vi "data2string.vi"(1 "Units":string="A", 2 "Numeric":dbl=0.0999646 format="%#_6p") -> (0 "resulting string":string="  99.964600   mA")   [LabVIEW 2013]
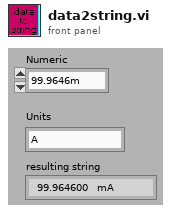
[diagram p1: front panel]
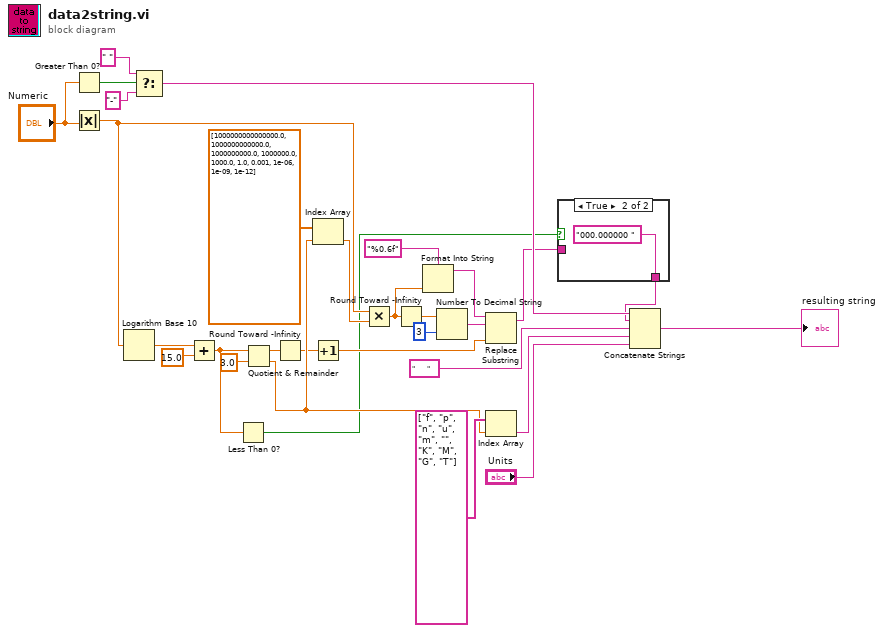
[diagram p0: block diagram]
diagram:
  n1 = Greater Than 0?(x="Numeric") -> (x > 0?=w13:bool)
  n2 = Absolute Value(x="Numeric") -> (abs(x)=w15:dbl)
  n3 = Logarithm Base 10(1:w15) -> (0:w28:dbl)
  n4 = Select(t=" ", s=w13, f="-") -> (s? t:f=w10:string)
  n5 = Add(x=w28, y=15.0) -> (x+y=w9:dbl)
  n6 = Less Than 0?(x=w9) -> (x < 0?=w1:bool)
  n7 = Quotient & Remainder(x=w9, y=3.0) -> (x-y*floor(x/y)=w21:dbl, floor(x/y)=w23:dbl)
  n8 = Round Toward -Infinity(1:w21) -> (0:w20:dbl)
  n9 = Index Array(array=dbl[] [1000000000000000.0, 1000000000000.0, 1000000000.0, 1000000.0, 1000.0, 1.0, 0.001, 1e-06, 1e-09, 1e-12], index=w23) -> (element=w25:dbl)
  n10 = Increment(x=w20) -> (x+1=w16:dbl)
  n11 = Multiply(x=w15, y=w25) -> (x*y=w6:dbl)
  n12 = Round Toward -Infinity(1:w6) -> (0:w7:dbl)
  n13 = Format Into String(format string="%0.6f", w6) -> (resulting string=w18:string)  [unwired: 2 in, 1 out]
  n14 = Number To Decimal String(number=w7, width (-)=i16 3) -> (decimal integer string=w19:string)
  n15 = Replace Substring(2:w16, 4:w19, 5:w18) -> (1:w3:string)  [unwired: 1 in, 1 out]
  n16 = Index Array(array=string[] ["f", "p", "n", "u", "m", "", "K", "M", "G", "T"], index=w23) -> (element=w17:string)
  n17 = case shown="True" w1 {
    tunnel: w3 -> [w31 _]
    tunnel: [w31 "000.000000 " ("format string")] -> w2
    frame False {
    }
    frame True {
    }
  }
  n18 = Concatenate Strings(w10, w2, "      " ("string"), w17, "Units") -> (→"resulting string":string)
